vi "encode_string (SubVI).vi"(10 "nsamp":i32, 11 "encode_string":string) -> (2 "encoded_cropped":bool[](array[boolean]), 3 "encoded_out":bool[](array[boolean]))   [LabVIEW 2022 SP3]
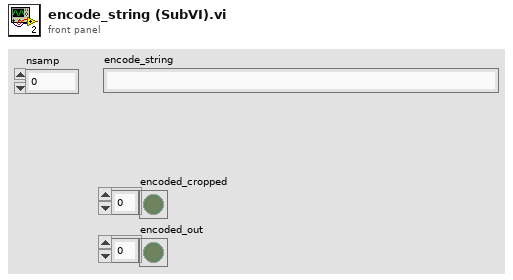
[diagram p1: front panel]
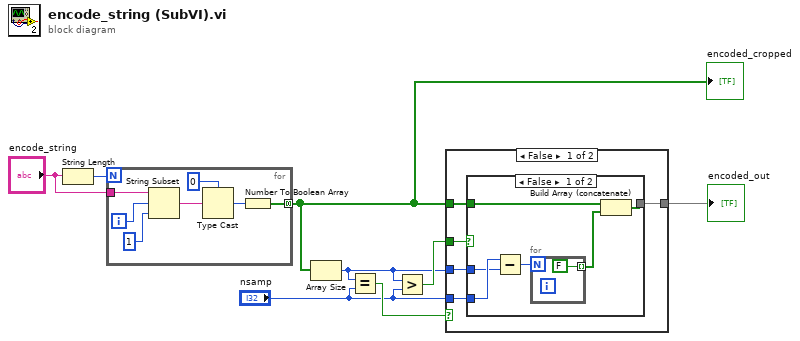
[diagram p0: block diagram]
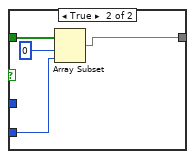
[diagram p2: hidden frame]
diagram:
  n1 = String Length(string="encode_string") -> (length=w8:i32)
  n2 = for {
    N: w8 -> [_]
    tunnel: "encode_string" -> [w15]
    tunnel: [w9] -> w1 mode=concatenating
    i -> [w14]
    n3 = String Subset(string=w15, offset (0)=w14, length (rest)=1 ("length (rest)")) -> (substring=w12:string)
    n4 = Type Cast(type=u8 0, x=w12) -> (*(type *) &x=w10:u8)
    n5 = Number To Boolean Array(number=w10) -> (Boolean array=w9:bool[])
  }
  "encoded_cropped" <- w1
  n6 = Array Size(array=w1) -> (size(s)=w3:i32)
  n7 = Equal?(x=w3, y="nsamp") -> (x = y?=w6:bool)
  n8 = Greater?(x=w3, y="nsamp") -> (0:w5:bool)
  n9 = case shown="False" w6 {
    tunnel: w1 -> [w19 w32]
    tunnel: [w18 w32] -> w2
    tunnel: w5 -> [w20 _]
    tunnel: "nsamp" -> [w17 _]
    tunnel: w3 -> [w16 _]
    frame False {
      n10 = case shown="False" w20 {
        tunnel: w19 -> [w26 w29]
        tunnel: [w21 w28] -> w18
        tunnel: w17 -> [w25 w30]
        tunnel: w16 -> [w24 _]
        frame False {
          n11 = Subtract(x=w25, y=w24) -> (x-y=w23:i32)
          n12 = for {
            N: w23 -> [_]
            tunnel: [FALSE] -> w22 mode=indexing
          }
          n13 = Build Array (concatenate)(w26, w22) -> (w21:bool[])
        }
        frame True {
          n14 = Array Subset(array=w29, index=0, length=w30) -> (w28:bool[])
        }
      }
    }
    frame True {
    }
  }
  "encoded_out" <- w2
